vi "Initialize Status Log Display.vi"(7 "QRD":T1, 8 "error in":errorcluster) -> (0 "error out":errorcluster, 5 "QRD Out":T1)   [LabVIEW 2025]
uses:
  Builds/Queue Wrappers.lvlibp/Q Packet.ctl
  Builds/Queue Wrappers.lvlibp
  Controls/Queues-Refs-Data.ctl
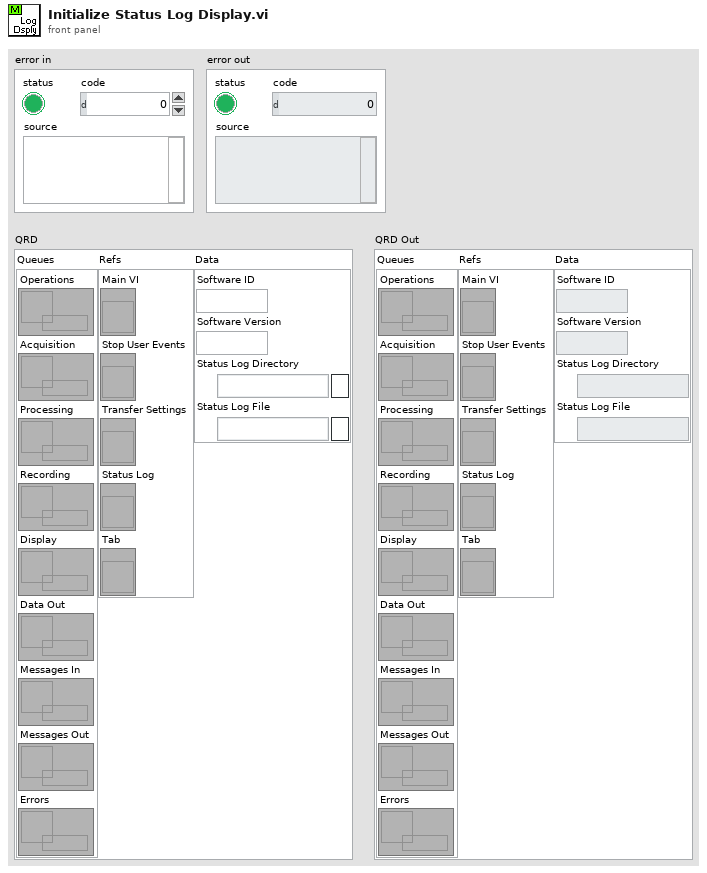
[diagram p1: front panel]
types:
  T1 = typedef "Queues-Refs-Data.ctl" = cluster{"Queues":cluster{"Operations":refnum<queue>, "Acquisition":refnum<queue>, "Processing":refnum<queue>, "Recording":refnum<queue>, "Display":refnum<queue>, "Data Out":refnum<queue>, "Messages In":refnum<queue>, "Messages Out":refnum<queue>, "Errors":refnum<queue>}, "Refs":cluster{"Main VI":refnum<vi>, "Stop User Events":refnum<vi>, "Transfer Settings":refnum<vi>, "Status Log":refnum<vi>, "Tab":refnum<vi>}, "Data":cluster{"Software ID":string, "Software Version":string, "Status Log Directory":path, "Status Log File":path}}
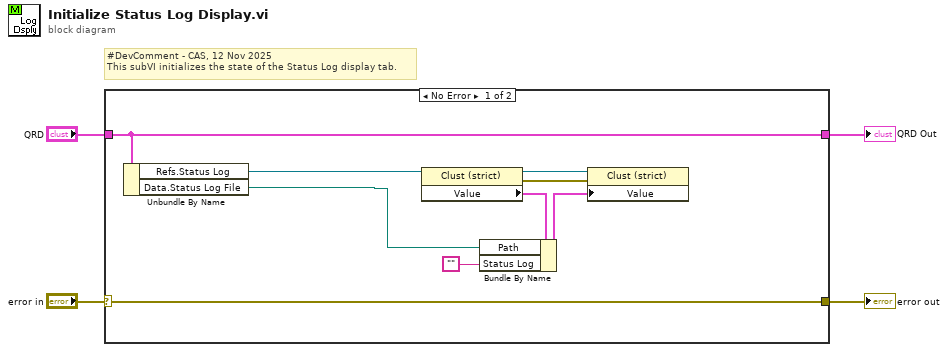
[diagram p0: block diagram]
diagram:
  # "#DevComment - CAS, 12 Nov 2025\nThis subVI initializes the state of the Status Log display tab."
  n1 = case shown="No Error" "error in" {
    selector: "error in" -> [w5 w14]
    tunnel: "QRD" -> [w6 w15]
    tunnel: [w6 w15] -> w3
    tunnel: [w5 w14] -> w1
    frame No Error {
      n2 = Unbundle By Name(w6) -> ("Refs.Status Log"=w13:refnum<vi>, "Data.Status Log File"=w9:path)
      n3 = property class="Clust (strict)"(reference=w13) -> (reference out=w12:refnum<vi>, error out=w11:errorcluster, "Value"=w10:cluster{"Status Log":string, "Path":path})  [unwired: 1 in]
      n4 = Bundle By Name(cluster=w10, "Path"=w9, "Status Log"="") -> (w7:cluster{"Status Log":string, "Path":path})
      n5 = property class="Clust (strict)"(reference=w12, error in=w11, "Value"=w7) -> ()  [unwired: 2 out]
    }
    frame Error {
    }
  }
  "error out" <- w1
  "QRD Out" <- w3
